vi "tb_acq_interp_simio.vi"() -> ()   [LabVIEW 2010]
uses:
  <vilib>/Platform/TimedLoop/XDataNode/XDataNode.xnode
  <vilib>/Platform/TimedLoop/XDataNode/timing_clust.ctl
  <vilib>/Platform/TimedLoop/XDataNode/nitl_modes.ctl
  <vilib>/Platform/TimedLoop/XDataNode/wakeup.ctl
  <vilib>/rvi/DataTransferAndStorage/Container/XNode/niFpgaContainer.xnode
  <vilib>/rvi/FXPMathLib/FxpInterpret/XNode/nifxpmath_Interpret.xnode
  Interpolation Block/Controls/Interpolation Input Data.ctl
  <vilib>/eio/EIONode/EIONode.xnode
  <vilib>/rvi/eio/nirviEIOImplementation/nirviEIOImplementation.xnode
  <vilib>/rvi/eio/common/nirviEmuClasses.ctl
  <vilib>/rvi/FIFO/Fifo_Resource/nirvififoEmulationSetSize.vi
  <vilib>/rvi/DataTransferAndStorage/Container/Common/niFpgaContainerGetUniqueNameForEmu.vi
  <vilib>/rvi/eio/common/nirviEmuTemplateMethod_noerrors.vi
  <vilib>/Platform/TimedLoop/XDataNode/XDNodeRunTimeDep.lvlib
panel:
  out "Resampled Data":i16(graph)
  in  "Write?":bool
  in  "Data":T1 {"x[n].ResampleInfo"."Lambda" format="%.18g"; "x[n-1].ResampleInfo"."Lambda" format="%.18g"}
  in  "Address":u32
  out "Interp Loop Overflow":bool
  out "acq timed out?":bool
  out "Numeric":i32
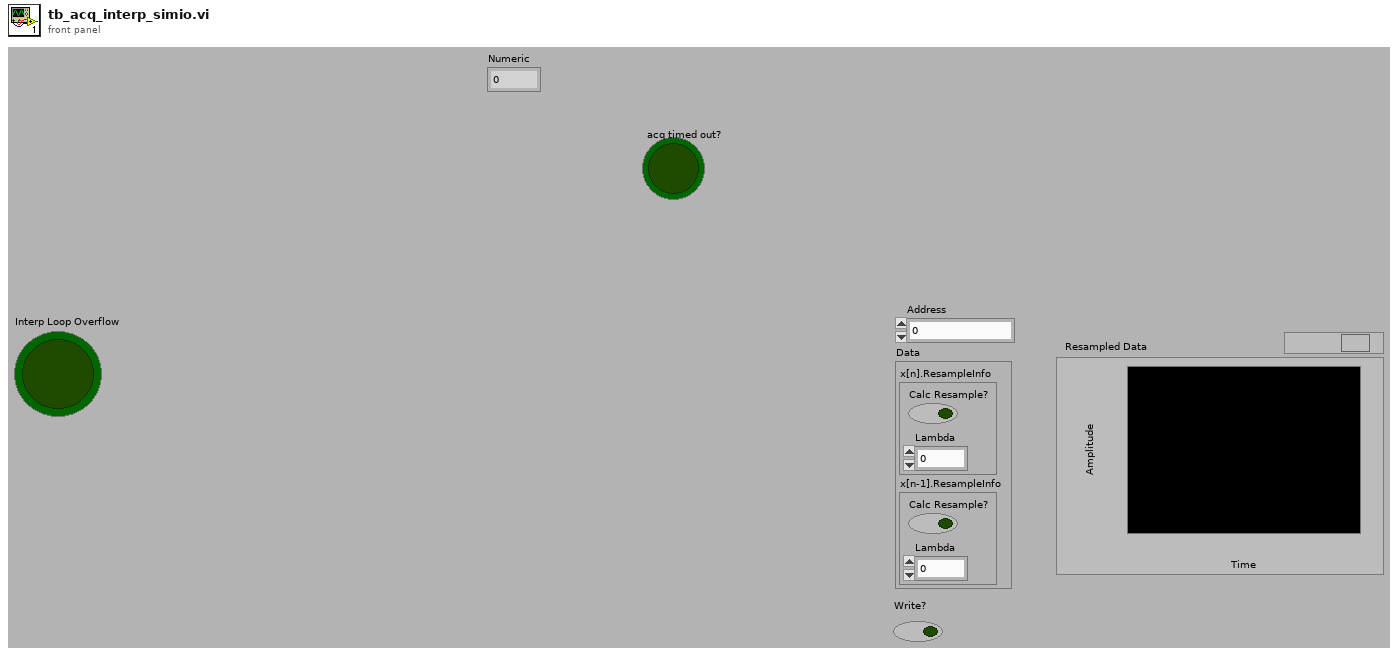
[diagram p1: front panel]
types:
  T1 = cluster{"x[n].ResampleInfo":cluster{"Calc Resample?":bool, "Lambda":fxp<+/-,18,1>}, "x[n-1].ResampleInfo":cluster{"Calc Resample?":bool, "Lambda":fxp<+/-,18,1>}}
  T2 = typedef "XDNodeRunTimeDep.lvlib/timing_clust.ctl" = cluster{"Expected End [f-1]":u64, "Actual End [f-1]":u64, "Finished Late? [f-1]":bool, "Expected End [i-1]":u64, "Actual End [i-1]":u64, "Finished Late? [i-1]":bool, "Expected Start [i]":u64, "Actual Start [i]":u64, "Expected Start [f]":u64, "Actual Start [f]":u64, "Source Name":string, "Structure Name":string, "Period":i64, "Deadline":i64, "Offset":i64, "Start":i64, "Priority":i32, "Timeout":i32, "Mode":T3, "Wakeup Reason":T4, "Error":errorcluster, "Source Type":string, "Secondary Source Type":string, "Global End Time":u64, "Global Start Time":u64, "Frame Duration":u64, "Iteration Duration":u64, "Assigned CPU":i32, "I/O Scan Engine Mode":u32}
  T3 = typedef "XDNodeRunTimeDep.lvlib/nitl_modes.ctl" = enum32{"No Change", "Process missed periods, maintain original phase", "Discard missed periods, maintain original phase", "Process missed periods, ignore original phase", "Discard missed periods, ignore original phase"}
  T4 = typedef "XDNodeRunTimeDep.lvlib/wakeup.ctl" = enum32{"Normal", "Aborted", "Asynchronous wakeup", "Timing source error", "Timed loop error", "Timeout"}
  T5 = typedef "Interpolation Input Data.ctl" = fxp<+/-,16,1>
  T6 = typedef "nirviEmuClasses.ctl" = enum16{"IO Read", "IO Write", "Method", "Property Read", "Property Write"}
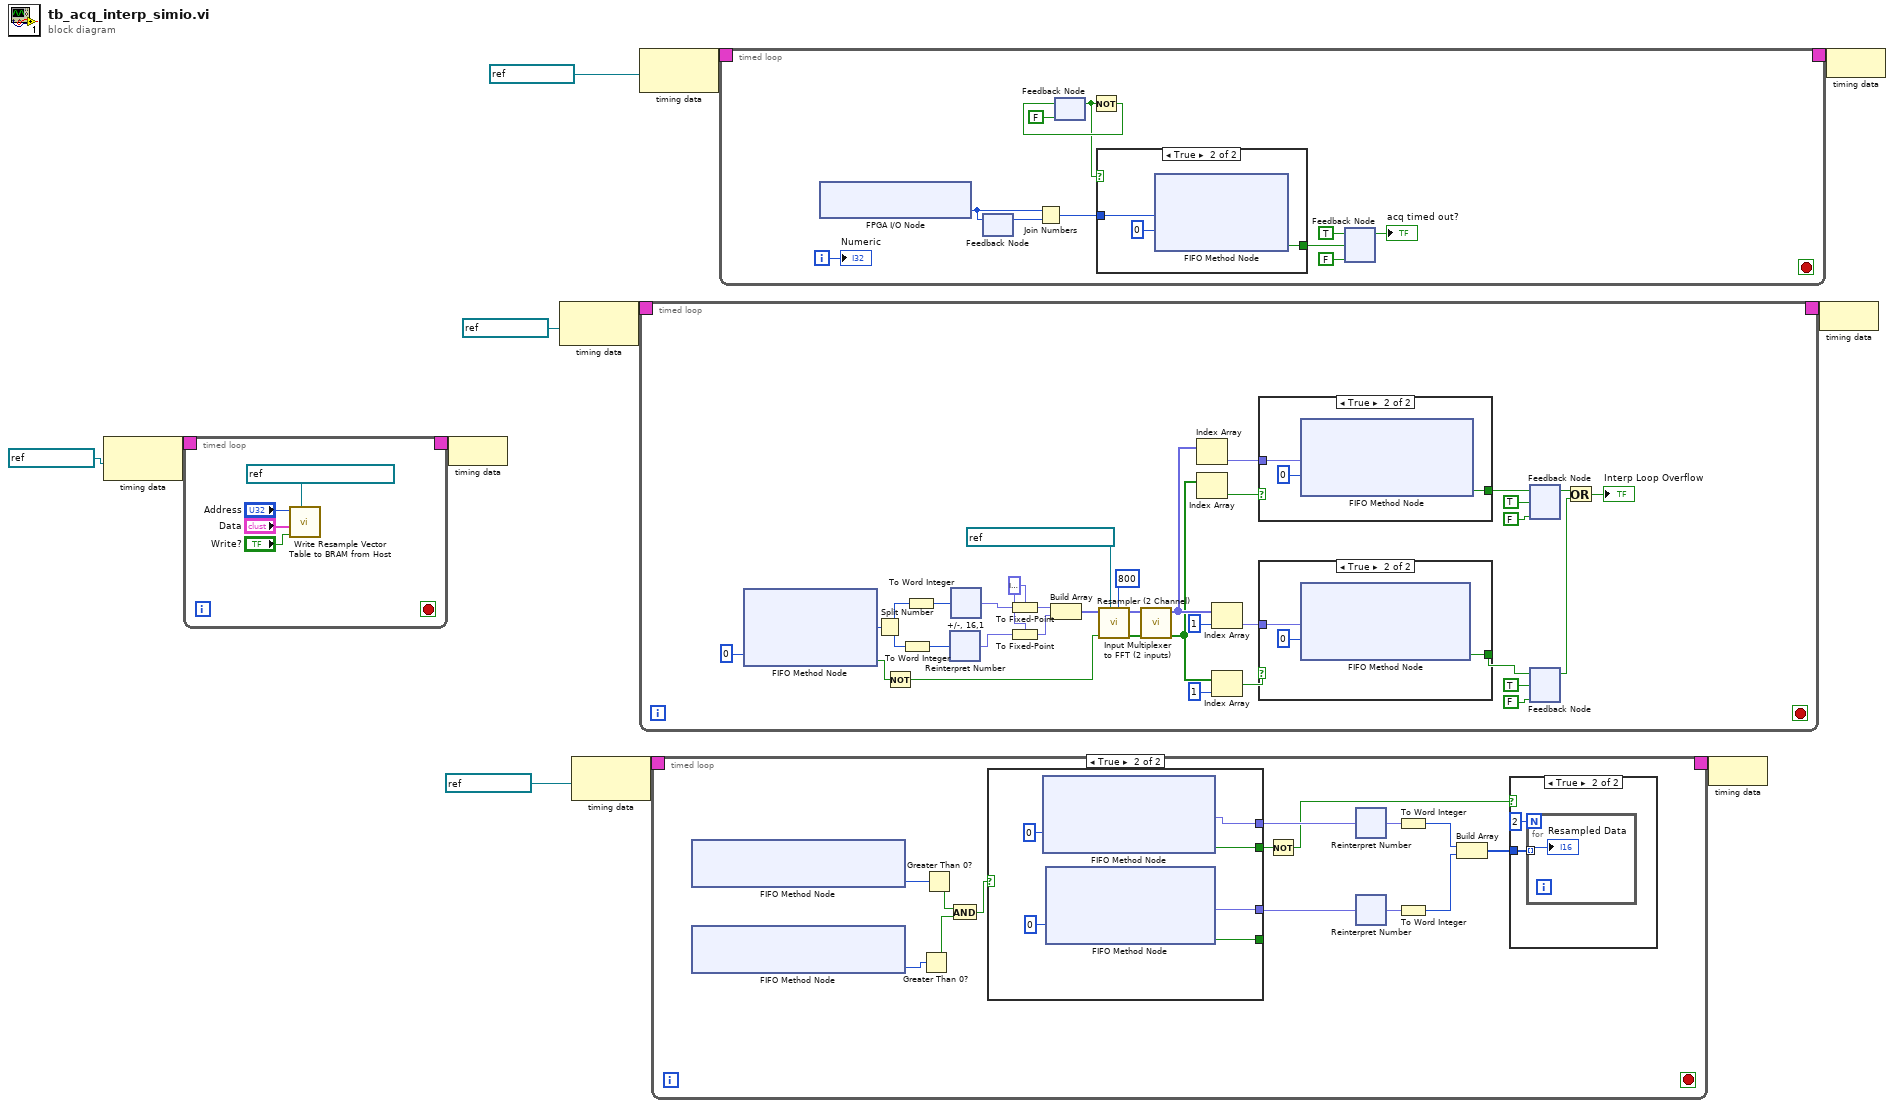
[diagram p0: block diagram]
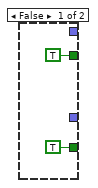
[diagram p3: hidden frame]
diagram:
  n1 = node-c288(refnum<k21> "126.67MHz" ("Source Name")) -> (w3:T2)
  n2 = timed-loop {
    timing: w3 -> [_]
    timing-out: [_] -> w2
    stop <- _ stop-if-true
    n3 = call "Write Resample Vector Table to BRAM from Host.vi"("Resample Table"=refnum<k21> "Resample Vector Table", "Write?"="Write?", "Data"="Data", "Address"="Address") -> ()  [unwired: 8 in]
  }
  n4 = node-c288(w2) -> ()
  n5 = node-c288(refnum<k21> "126.67MHz" ("Source Name")) -> (w10:T2)
  n6 = node-c288(refnum<k21> "126.67MHz" ("Source Name")) -> (w8:T2)
  n7 = node-c288(refnum<k21> "ADC Clock" ("Source Name")) -> (w12:T2)
  n8 = timed-loop {
    timing: w10 -> [_]
    timing-out: [_] -> w9
    stop <- _ stop-if-true
    w31 = T5 0.0 ("Interpolate.Input Data")
    n9 = xnode ("FIFO Method Node")("Timeout"=0) -> ("Element"=w34:u32, "Timed Out?"=w29:bool)  [unwired: 1 in, 1 out]
    n10 = Split Number(x=w34) -> (hi(x)=w27:u16, lo(x)=w26:u16)
    n11 = Not(x=w29) -> (.not. x?=w24:bool)
    n12 = To Word Integer(number=w26) -> (16bit integer=w22:i16)
    n13 = To Word Integer(number=w27) -> (16bit integer=w21:i16)
    n14 = xnode "Reinterpret Number"("x"=w22) -> ("y"=w25:fxp<+/-,16,1>)
    n15 = xnode "+/-, 16,1"("x"=w21) -> ("y"=w20:fxp<+/-,16,1>)
    n16 = To Fixed-Point(fixed-point type=w31, number=w20) -> (fixed-point=w23:T5)
    n17 = To Fixed-Point(fixed-point type=w31, number=w25) -> (fixed-point=w32:T5)
    n18 = Build Array(w23, w32) -> (w30:T5[])
    n19 = call "Resampler (2 Channel).vi"("CalibrationTable Length-1"=u16 800, "ResampleVectorInfo"=refnum<k21> "Resample Vector Table", "DataValid"=w24, "Input Data"=w30) -> ("Data Valid"=w52:bool[], "Interpolated Data"=w53:T5[])  [unwired: 6 in]
    n20 = call "Input Multiplexer to FFT (2 inputs).vi"("Input Data Valid Array"=w52, "Input Data"=w53) -> ("Output Data Valid Array"=w47:bool[], "Interchanged Data"=w49:fxp<+/-,16,1>[])  [unwired: 8 in]
    n21 = Index Array(array=w49) -> (element=w51:fxp<+/-,16,1>)  [unwired: 1 in]
    n22 = Index Array(array=w47) -> (element=w50:bool)  [unwired: 1 in]
    n23 = Index Array(array=w49, index=1) -> (element=w48:fxp<+/-,16,1>)
    n24 = Index Array(array=w47, index=1) -> (element=w46:bool)
    n25 = case shown="True" w50 {
      tunnel: w51 -> [_ w165]
      tunnel: [_ w163] -> w43
      frame False {
      }
      frame True {
        n26 = xnode ("FIFO Method Node")("Element"=w165, "Timeout"=0) -> ("Timed Out?"=w163:bool)  [unwired: 1 in, 1 out]
      }
    }
    n27 = case shown="True" w46 {
      tunnel: w48 -> [_ w111]
      tunnel: [_ w109] -> w40
      frame False {
      }
      frame True {
        n28 = xnode ("FIFO Method Node")("Element"=w111, "Timeout"=0) -> ("Timed Out?"=w109:bool)  [unwired: 1 in, 1 out]
      }
    }
    n29 = feedback-in #1(w43, TRUE) -> ()
    n30 = feedback #1(FALSE ("Timed Out?")) -> (w39:bool)
    n31 = feedback #2(FALSE ("Timed Out?")) -> (w36:bool)
    n32 = feedback-in #2(w40, TRUE) -> ()
    n33 = Or(x=w39, y=w36) -> (x .or. y?=→"Interp Loop Overflow":bool)
  }
  n34 = timed-loop {
    timing: w8 -> [_]
    timing-out: [_] -> w7
    stop <- _ stop-if-true
    n35 = xnode ("FIFO Method Node")() -> ("Number of Elements to Read"=w225:u32)  [unwired: 1 in, 1 out]
    n36 = xnode ("FIFO Method Node")() -> ("Number of Elements to Read"=w229:u32)  [unwired: 1 in, 1 out]
    n37 = Greater Than 0?(x=w229) -> (x > 0?=w227:bool)
    n38 = Greater Than 0?(x=w225) -> (x > 0?=w228:bool)
    n39 = And(x=w228, y=w227) -> (x .and. y?=w226:bool)
    n40 = case shown="True" w226 {
      tunnel: [TRUE ("Timed Out?") w294] -> w232
      tunnel: [_ w293] -> w231
      tunnel: [_ w292] -> w230
      tunnel: [TRUE ("Timed Out?") w291] -> _
      frame False {
      }
      frame True {
        n41 = xnode ("FIFO Method Node")("Timeout"=0) -> ("Element"=w293:fxp<+/-,16,1>, "Timed Out?"=w294:bool)  [unwired: 1 in, 1 out]
        n42 = xnode ("FIFO Method Node")("Timeout"=0) -> ("Element"=w292:fxp<+/-,16,1>, "Timed Out?"=w291:bool)  [unwired: 1 in, 1 out]
      }
    }
    n43 = Not(x=w232) -> (.not. x?=w219:bool)
    n44 = xnode "Reinterpret Number"("x"=w231) -> ("y"=w224:fxp<+/-,16,16>)
    n45 = xnode "Reinterpret Number"("x"=w230) -> ("y"=w223:fxp<+/-,16,16>)
    n46 = To Word Integer(number=w224) -> (16bit integer=w222:i16)
    n47 = To Word Integer(number=w223) -> (16bit integer=w221:i16)
    n48 = Build Array(w222, w221) -> (w220:i16[])
    n49 = case shown="True" w219 {
      tunnel: w220 -> [_ w234]
      frame False {
      }
      frame True {
        n50 = for {
          N: 2 -> [_]
          tunnel: w234 -> [w235] mode=indexing
          "Resampled Data" <- w235
        }
      }
    }
  }
  n51 = timed-loop {
    timing: w12 -> [_]
    timing-out: [_] -> w11
    i -> [w446]
    stop <- _ stop-if-true
    n52 = xnode "FPGA I/O Node"() -> ("IO Module\\AI 0 Data"=w454:i16)  [unwired: 1 in, 1 out]
    n53 = feedback-in #3(w454) -> ()
    n54 = feedback #3() -> (w453:i16)  [unwired: 1 in]
    n55 = Join Numbers(hi=w454, lo=w453) -> ((hi.lo)=w444:u32)
    n56 = feedback #4(FALSE) -> (w445:bool)
    n57 = Not(x=w445) -> (.not. x?=w452:bool)
    n58 = feedback-in #4(w452) -> ()
    n59 = case shown="True" w445 {
      tunnel: w444 -> [_ w457]
      tunnel: [_ w455] -> w449
      frame False {
      }
      frame True {
        n60 = xnode ("FIFO Method Node")("Element"=w457, "Timeout"=0) -> ("Timed Out?"=w455:bool)  [unwired: 1 in, 1 out]
      }
    }
    n61 = feedback-in #5(TRUE, w449) -> ()
    n62 = feedback #5(FALSE) -> (→"acq timed out?":bool)
    "Numeric" <- w446
  }
  n63 = node-c288(w7) -> ()
  n64 = node-c288(w9) -> ()
  n65 = node-c288(w11) -> ()
